vi "Generate Trace for Received Message.vi"(9 "Actor":refnum<class "Message Enqueuer.lvclass">, 10 "Message Name":string) -> ()   [LabVIEW 2020, in "Actor Framework.lvlib"]
doc: "Generates a DETT User Generated Trace for a message object being received by an actor."
uses:
  vi.lib/ActorFramework/Actor Framework.lvlib
  vi.lib/ActorFramework/Message Enqueuer/Message Enqueuer.lvclass
  vi.lib/ActorFramework/tracing/Support/Registration Mode.ctl
  vi.lib/ActorFramework/tracing/Support/Localized Strings.vi
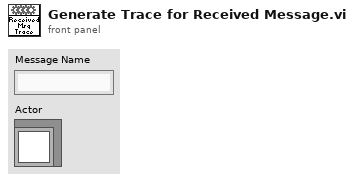
[diagram p1: front panel]
types:
  T1 = typedef "Actor Framework.lvlib/Registration Mode.ctl" = enum16{"Register Actor", "Get ID", "Get Enqueuer", "Deregister Actor", "Get Update Event", "Get All Actors", "Set Actor Core Name"}
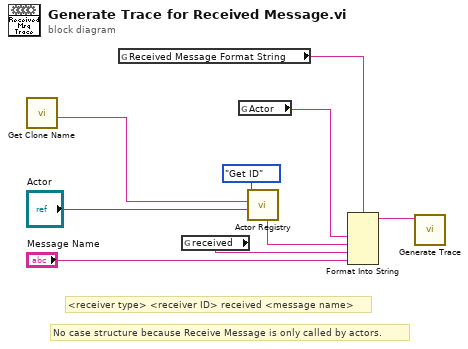
[diagram p0: block diagram]
diagram:
  # "No case structure because Receive Message is only called by actors."
  # "<receiver type> <receiver ID> received <message name>"
  n1 = call "Get Clone Name.vi"() -> ("Clone ID"=w4:string)  [unwired: 10 in, 1 out]
  n2 = global read "Localized Strings.vi" "Received Message Format String"() -> (w3:string)
  n3 = global read "Localized Strings.vi" "received"() -> (w2:string)
  n4 = global read "Localized Strings.vi" "Actor"() -> (w8:string)
  n5 = call "Actor Registry.vi"("Actor Enqueuer"="Actor", "Actor ID"=w4, "Action"=Registration_Mode."Get ID") -> ("Actor Alias out"=w7:string)  [unwired: 4 in, 4 out]
  n6 = Format Into String(format string=w3, w8, w7, w2, "Message Name") -> (resulting string=w1:string)  [unwired: 2 in, 1 out]
  n7 = call "Generate Trace.vi"("String"=w1) -> ()  [unwired: 11 in]
